vi "Set Label Properties.vi"(8 "error in":errorcluster, 10 "label properties":T1, 11 "label ref":T3 format="%.0x") -> (0 "error out":errorcluster, 3 "label ref out":T3 format="%.0x")   [LabVIEW 2020, in "AIM ARINC 429 Scripting.lvlib"]
uses:
  <vilib>/NI VeriStand/Custom Device API/Custom Device Item Ref.ctl
  Shared/Label Properties.ctl
  Shared/Label.ctl
  Constants.vi
  <vilib>/NI VeriStand/Custom Device API/Set Item Property (I32).vi
  <vilib>/NI VeriStand/Custom Device API/Set Item Property (U16).vi
  <vilib>/NI VeriStand/Custom Device API/Set Item Property (Boolean).vi
  AIM ARINC 429 Scripting.lvlib
  <vilib>/NI VeriStand/Custom Device API/Custom Device API.lvlib
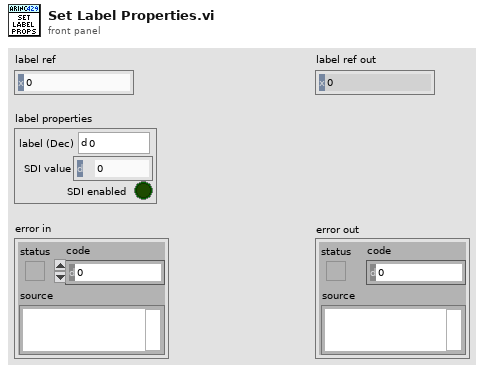
[diagram p1: front panel]
types:
  T1 = typedef "Label Properties.ctl" = cluster{"label (Dec)":T2, "SDI value":u8, "SDI enabled":bool}
  T2 = typedef "Label.ctl" = u8
  T3 = typedef "Custom Device API.lvlib/Custom Device Item Ref.ctl" = u64
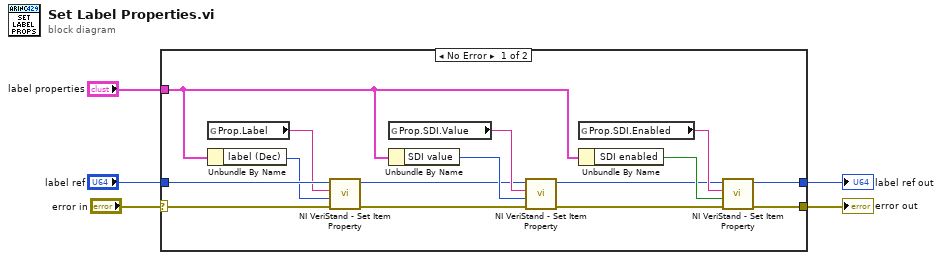
[diagram p0: block diagram]
diagram:
  n1 = case shown="No Error" "error in" {
    selector: "error in" -> [w19 w22]
    tunnel: [w7 w22] -> w4
    tunnel: "label ref" -> [w20 w21]
    tunnel: [w8 w21] -> w2
    tunnel: "label properties" -> [w6 _]
    frame No Error {
      n2 = global read "Constants.vi" "Prop.Label"() -> (w18:string)
      n3 = Unbundle By Name(w6) -> ("label (Dec)"=w17:T2)
      n4 = call-poly <vilib>:"NI VeriStand - Set Item Property.vi"("error in (no error)"=w19, "Value"=w17, "Property Name"=w18, "Item Ref in"=w20) -> ("error out"=w14:errorcluster, "Item Ref out"=w13:T3)  [unwired: 5 in, 1 out]
      n5 = global read "Constants.vi" "Prop.SDI.Value"() -> (w15:string)
      n6 = Unbundle By Name(w6) -> ("SDI value"=w16:u8)
      n7 = call-poly <vilib>:"NI VeriStand - Set Item Property.vi"("error in (no error)"=w14, "Value"=w16, "Property Name"=w15, "Item Ref in"=w13) -> ("error out"=w9:errorcluster, "Item Ref out"=w10:T3)  [unwired: 5 in, 1 out]
      n8 = global read "Constants.vi" "Prop.SDI.Enabled"() -> (w12:string)
      n9 = Unbundle By Name(w6) -> ("SDI enabled"=w11:bool)
      n10 = call-poly <vilib>:"NI VeriStand - Set Item Property.vi"("error in (no error)"=w9, "Value"=w11, "Property Name"=w12, "Item Ref in"=w10) -> ("error out"=w7:errorcluster, "Item Ref out"=w8:T3)  [unwired: 5 in, 1 out]
    }
    frame Error {
    }
  }
  "label ref out" <- w2
  "error out" <- w4
